vi "How to Build Coefficients Quantizer.vi"() -> ()   [LabVIEW 2023]
doc: "Demonstrates how to use the DFD Convert FXP to Integer VI and the DFD Convert Integer to FXP VI to build a quantizer from a group of coefficients.\n\nExamine the block diagram to learn how to build a quantizer for a group of coefficients."
uses:
  <vilib>/addons/Digital Filter Design/_Objects.llb/DFD Quantization Settings.ctl
  <vilib>/addons/Digital Filter Design/_Objects.llb/DFD Quantization Sources.ctl
  <vilib>/addons/Digital Filter Design/FXPLib.llb/DFD FXP to I32 (vector).vi
  <vilib>/addons/Digital Filter Design/FXPLib.llb/DFD I32 to FXP (vector).vi
  <vilib>/addons/Digital Filter Design/NI_DigFilterLicensed.lvlib
panel:
  in  "Coefficients Word Length":i16=16
  out "Coefficients Quantizer":T1={"source"=7, "wl"=16, "iwl"=1, "overflow mode"=enum."Wrap", "rounding mode"=enum."Truncation", "signed?"=TRUE} {"source" items=["Coefficients a/k"=0, "Coefficients b/v"=7, "Input"=1, "Output"=2, "Multiplicand"=3, "Product"=4, "Sum"=5, "Delay"=6]}
  out "Integer Coefficients":i32[](array[numeric])
  out "Fixed-Point Coefficients":dbl[](array[numeric])
  in  "Floating-Point Coefficients":dbl[](array[numeric])=[0.5, 0.5]
  # "Select Help>>Show Context Help and move the cursor over the VI icon for more information."
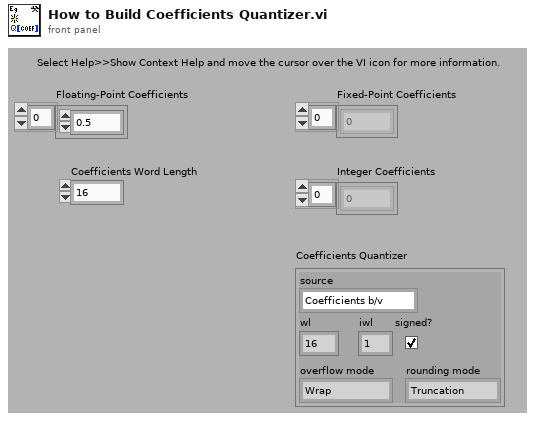
[diagram p1: front panel]
types:
  T1 = typedef "NI_DigFilterLicensed.lvlib/DFD Quantization Settings.ctl" = cluster{"source":T2, "wl":i16, "iwl":i16, "overflow mode":enum16{"Saturation", "Wrap"}, "rounding mode":enum16{"Nearest", "Truncation"}, "signed?":bool}
  T2 = typedef "NI_DigFilterLicensed.lvlib/DFD Quantization Sources.ctl" = u16
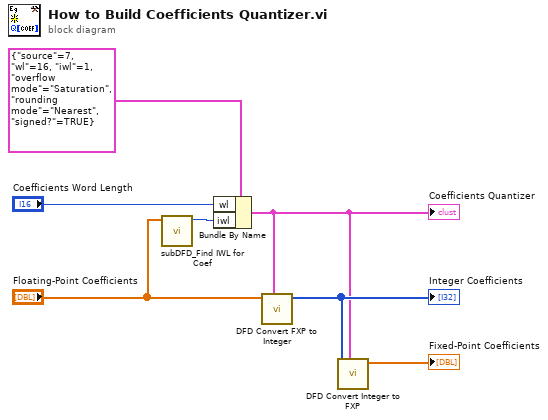
[diagram p0: block diagram]
diagram:
  n1 = call <vilib>:"subDFD_Find IWL for Coef.vi"("coefficients"="Floating-Point Coefficients") -> ("iwl"=w5:i16)  [unwired: 10 out]
  n2 = Bundle By Name(cluster=T1 {"source"=7, "wl"=16, "iwl"=1, "overflow mode"=enum."Saturation", "rounding mode"=enum."Nearest", "signed?"=TRUE} ("coefficients quantizer"), "wl"="Coefficients Word Length", "iwl"=w5) -> (w2:T1)
  "Coefficients Quantizer" <- w2
  n3 = call-poly <vilib>:"DFD Convert FXP to Integer.vi"("quantization settings"=w2, "FXP values"="Floating-Point Coefficients") -> ("I32 values"=w3:i32[])  [unwired: 1 in, 8 out]
  "Integer Coefficients" <- w3
  n4 = call-poly <vilib>:"DFD Convert Integer to FXP.vi"("quantization settings"=w2, "I32 values"=w3) -> ("FXP values"=→"Fixed-Point Coefficients":dbl[])  [unwired: 1 in, 8 out]
